vi "Set VI Icon.vi"(8 "error in (no error)":errorcluster, 10 "Icon":refnum<class "Icon.lvclass">, 11 "VI Refnum in":refnum<vi>) -> (0 "error out":errorcluster, 3 "VI Refnum out":refnum<vi>)   [LabVIEW 2017, in "LabVIEW Icon API.lvlib"]
doc: "Specifies the LabVIEW Icon class of a VI."
uses:
  <vilib>/LabVIEW Icon API/LabVIEW Icon API.lvlib
  <vilib>/LabVIEW Icon API/lv_icon/Classes/Icon/Icon.lvclass
  <vilib>/LabVIEW Icon API/lv_icon/lv_icon.lvlib
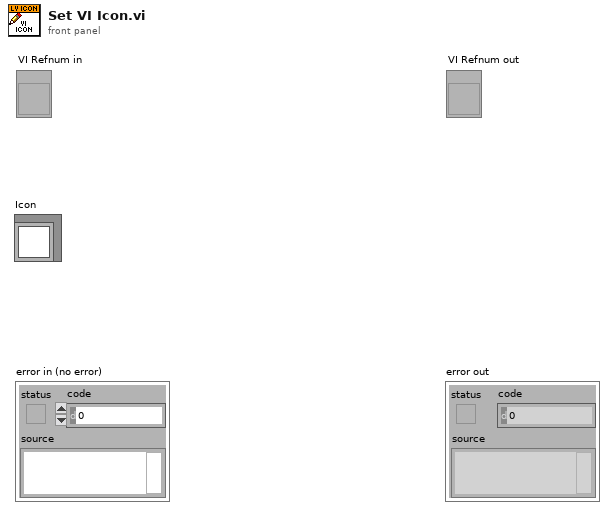
[diagram p1: front panel]
types:
  T1 = typedef "imagedata.ctl" = cluster{"image type":i32, "image depth":i32, "image":u8[], "mask":u8[], "colors":u32[], "Rectangle":cluster{"left":i16, "top":i16, "right":i16, "bottom":i16}}
  T2 = typedef "LabVIEW Icon Stored Information.ctl" = cluster{"Text Visible?":bool, "Text Opacity":u8, "Templ Visible?":bool, "Templ Opacity":u8, "Relative Path from 1 to 2":path, "Image":picture, "All User Layers":refnum<class "Layer.lvclass">[], "Body Text":T3}
  T3 = typedef "BodyText.ctl" = cluster{"Line 1 text":string, "Line 2 text":string, "Line 3 text":string, "Line 4 text":string, "Line 1 color":u32, "Line 2 color":u32, "Line 3 color":u32, "Line 4 color":u32, "Body Text Spec":cluster{"Font":T4, "Alignment":T5, "Size":u8}, "Center text vertically":bool, "Capitalize Text":bool}
  T4 = typedef "Font.ctl" = string
  T5 = typedef "Alignment.ctl" = u16
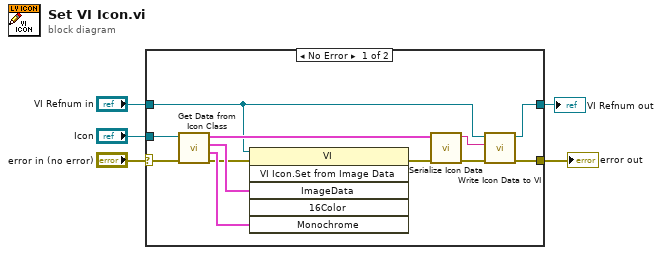
[diagram p0: block diagram]
diagram:
  n1 = case shown="No Error" "error in (no error)" {
    selector: "error in (no error)" -> [w17 w19]
    tunnel: [w6 w19] -> w2
    tunnel: [w8 w18] -> w3
    tunnel: "VI Refnum in" -> [w9 w18]
    tunnel: "Icon" -> [w16 _]
    frame No Error {
      n2 = call <vilib>:"Get Data from Icon Class.vi"("error in (no error)"=w17, "Icon in"=w16) -> ("error out"=w13:errorcluster, "BW Image Data"=w14:T1, "Color Image Data"=w15:T1, "Icon data"=w12:T2)  [unwired: 6 in]
      n3 = invoke class="VI" method="VI Icon.Set from Image Data"(reference=w9, error in=w13, "ImageData"=w15, "Monochrome"=w14) -> (error out=w11:errorcluster)  [unwired: 2 in, 5 out]
      n4 = call <vilib>:"Serialize Icon Data.vi"("error in"=w11, "Icon data"=w12) -> ("error out"=w10:errorcluster, "data string"=w7:string)  [unwired: 8 in]
      n5 = call <vilib>:"Write Icon Data to VI.vi"("error in (no error)"=w10, "Data"=w7, "VI Ref in"=w9) -> ("error out"=w6:errorcluster, "VI Ref out"=w8:refnum<vi>)  [unwired: 7 in]
    }
    frame Error {
    }
  }
  "error out" <- w2
  "VI Refnum out" <- w3
